vi "ClearTreeControls (SubVI).vi"(8 "error in (no error)":errorcluster, 11 "Tree Control Refnums":refnum<vi>[](array[refnum])) -> (0 "error out":errorcluster)   [LabVIEW 2018, in "MainFrameLib.lvlib"]
uses:
  MainFrameLib.lvlib
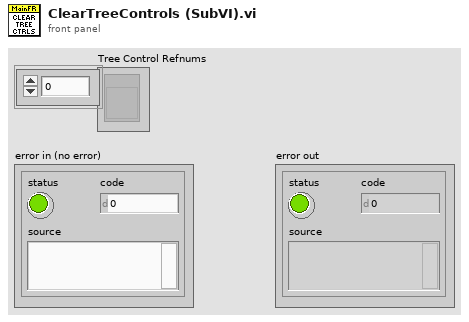
[diagram p1: front panel]
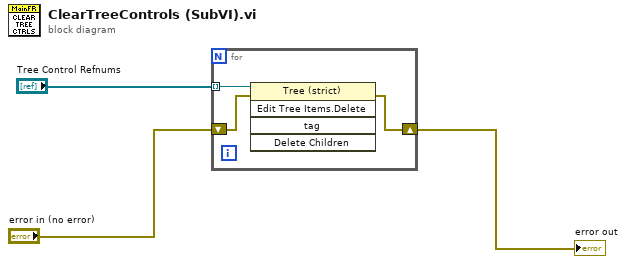
[diagram p0: block diagram]
diagram:
  n1 = for {
    tunnel: "Tree Control Refnums" -> [w6] mode=indexing
    shift-right: [w5] -> w1
    shift-left: "error in (no error)" -> [w4]
    n2 = invoke on="Invoke Node" class="Tree (strict)" method="Edit Tree Items.Delete"(reference=w6, error in=w4) -> (error out=w5:errorcluster)  [unwired: 3 in, 4 out]
  }
  "error out" <- w1
